vi "rsscope_FormatUSBPDPacketTypeInt32_WriteCallback.vi"(5 "Attribute":T1={"Identifier"="", "Descriptive Name"="", "Data Type"=enum."Integer 32", "Command"="", "Access"=enum."Read/Write", "Range Table"="", "Read Callback"="", "Write Callback"="", "Supported Models"="", "Instrument Options"="", "Index"=0, "OPC Wait"=FALSE, "No Status Check"=FALSE, "Cache Only"=FALSE}, 7 "Repeated Capability":string, 8 "error in (no error)":errorcluster, 10 "Attribute Value I32":i32, 11 "VISA resource name":refnum<visa-resource-name>) -> (0 "error out":errorcluster, 3 "VISA resource name out":refnum<visa-resource-name>)   [LabVIEW 2018]
doc: "This VI sets the attribute value.\n\nThis is a low-level VI that you can use to set the values of instrument-specific properties and inherent IVI properties. If the property represents an instrument state, this VI performs instrument I/O in the following cases:\n\n- State caching is disabled for the entire session or for the particular property.\n\n- State caching is enabled and the currently cached value is invalid or is different than the value you specify. \n\nThis instrument driver contains high-level VIs that set most of the instrument properties. It is best to use the high-level driver VIs as much as possible. They handle order dependencies and multithread locking for you. In addition, they perform status checking only after setting all of the properties. In contrast, when you set multiple properties using the SetAttribute VIs, the VIs check the instrument status after each call.\n\nAlso, when state caching is enabled, the high-level VIs that configure multiple properties perform instrument I/O only for the properties whose value you change. Thus, you can safely call the high-level VIs without the penalty of redundant instrument I/O."
uses:
  rsidr_core.llb/type_Attribute.ctl
  rsidr_core.llb/type_Attribute_Data_Type.ctl
  rsidr_core.llb/type_ReadWriteAccess.ctl
  rsidr_core.llb/rsscope_rsidr_core.lvlib
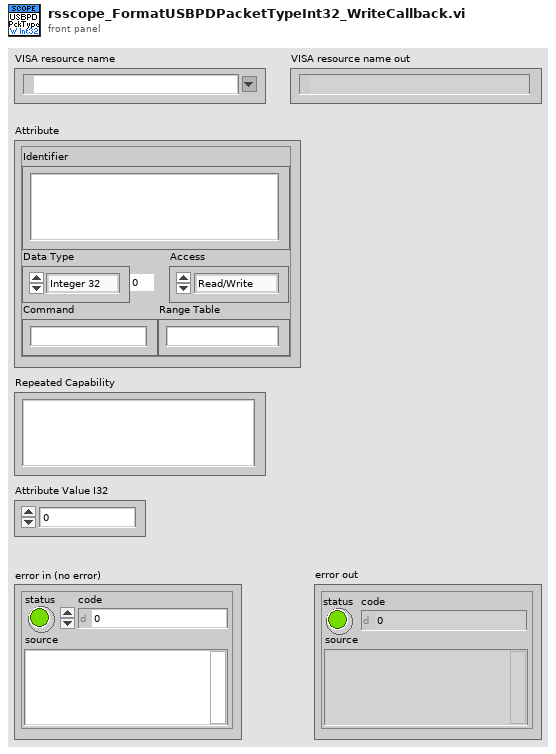
[diagram p1: front panel]
types:
  T1 = typedef "rsscope_rsidr_core.lvlib/type_Attribute.ctl" = cluster{"Identifier":string, "Descriptive Name":string, "Data Type":T2, "Command":string, "Access":T3, "Range Table":string, "Read Callback":string, "Write Callback":string, "Supported Models":string, "Instrument Options":string, "Index":i32, "OPC Wait":bool, "No Status Check":bool, "Cache Only":bool}
  T2 = typedef "rsscope_rsidr_core.lvlib/type_Attribute_Data_Type.ctl" = enum16{"Integer 32", "Double", "String", "Boolean", "None", "Integer 64", "RawString"}
  T3 = typedef "rsscope_rsidr_core.lvlib/type_ReadWriteAccess.ctl" = enum16{"Read Only", "Write Only", "Read/Write"}
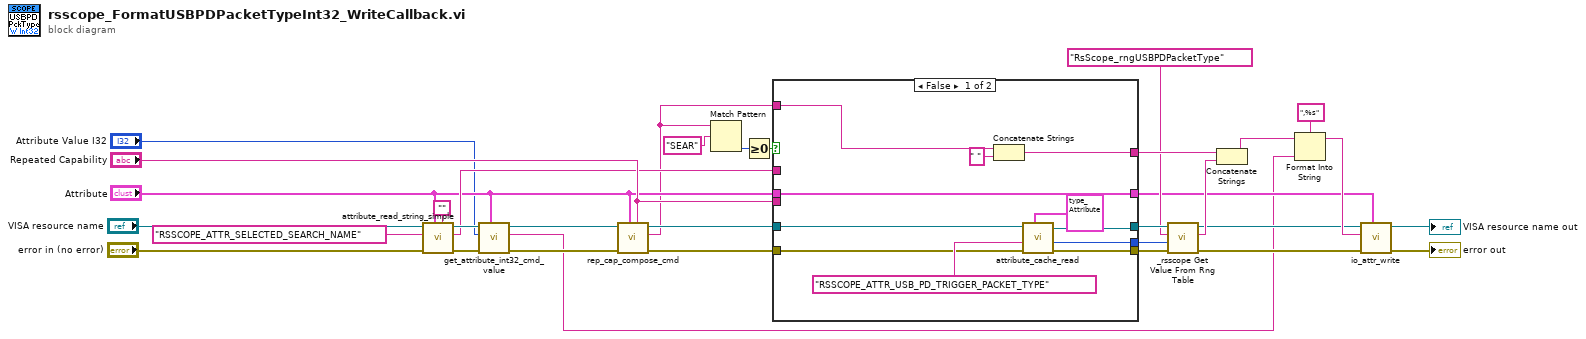
[diagram p0: block diagram]
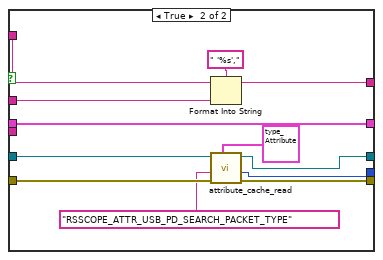
[diagram p2: hidden frame]
diagram:
  n1 = call "attribute_read_string_simple.vi"("Repeated Capability"="" ("Empty String Constant"), "Attribute"="Attribute", "error in"="error in (no error)", "Direct Attribute ID (\"\")"="RSSCOPE_ATTR_SELECTED_SEARCH_NAME" ("Direct Attribute ID (\"\")"), "VISA resource name"="VISA resource name") -> ("error out"=w27:errorcluster, "String out"=w8:string, "VISA resource name out"=w26:refnum<visa-resource-name>)  [unwired: 4 in]
  n2 = call "get_attribute_int32_cmd_value.vi"("Attribute"="Attribute", "error in"=w27, "Input Int32 value"="Attribute Value I32", "VISA resource name"=w26) -> ("error out"=w25:errorcluster, "Cmd Value out"=w1:string, "VISA resource name out"=w24:refnum<visa-resource-name>)  [unwired: 5 in]
  n3 = call "rep_cap_compose_cmd.vi"("Repeated Capability"="Repeated Capability", "Attribute"="Attribute", "error in"=w25, "VISA resource name"=w24) -> ("error out"=w13:errorcluster, "Command out"=w3:string, "VISA resource name out"=w12:refnum<visa-resource-name>)  [unwired: 5 in]
  n4 = Match Pattern(string=w3, regular expression="SEAR" ("true string")) -> (offset past match=w16:i32)  [unwired: 1 in, 3 out]
  n5 = Greater Or Equal To 0?(x=w16) -> (x >= 0?=w15:bool)
  n6 = case shown="False" w15 {
    tunnel: w8 -> [_ w55]
    tunnel: [w44 w54] -> w22
    tunnel: w3 -> [w34 w53]
    tunnel: w12 -> [w38 w49]
    tunnel: w13 -> [w39 w50]
    tunnel: [w36 w48] -> w21
    tunnel: [w37 w47] -> w20
    tunnel: [w35 w46] -> w19
    tunnel: "Repeated Capability" -> [_ _]
    tunnel: "Attribute" -> [w42 w52]
    tunnel: [w42 w52] -> w6
    frame False {
      n7 = Concatenate Strings(w34, " " ("string")) -> (w44:string)
      n8 = call "attribute_cache_read.vi"("Attribute"=T1 {"Identifier"="", "Descriptive Name"="", "Data Type"=enum."Integer 32", "Command"="", "Access"=enum."Read/Write", "Range Table"="", "Read Callback"="", "Write Callback"="", "Supported Models"="", "Instrument Options"="", "Index"=0, "OPC Wait"=FALSE, "No Status Check"=FALSE, "Cache Only"=FALSE}, "error in"=w39, "Direct Attribute ID (Attribute cluster)"="RSSCOPE_ATTR_USB_PD_TRIGGER_PACKET_TYPE" ("Direct Attribute ID (\"\")"), "VISA resource name"=w38) -> ("error out"=w37:errorcluster, "Int32 out"=w35:i32, "VISA resource name out"=w36:refnum<visa-resource-name>)  [unwired: 5 out]
    }
    frame True {
      n9 = Format Into String(format string=" '%s',", initial string=w53, w55) -> (resulting string=w54:string)  [unwired: 1 in, 1 out]
      n10 = call "attribute_cache_read.vi"("Attribute"=T1 {"Identifier"="", "Descriptive Name"="", "Data Type"=enum."Integer 32", "Command"="", "Access"=enum."Read/Write", "Range Table"="", "Read Callback"="", "Write Callback"="", "Supported Models"="", "Instrument Options"="", "Index"=0, "OPC Wait"=FALSE, "No Status Check"=FALSE, "Cache Only"=FALSE}, "error in"=w50, "Direct Attribute ID (Attribute cluster)"="RSSCOPE_ATTR_USB_PD_SEARCH_PACKET_TYPE" ("Direct Attribute ID (\"\")"), "VISA resource name"=w49) -> ("error out"=w47:errorcluster, "Int32 out"=w46:i32, "VISA resource name out"=w48:refnum<visa-resource-name>)  [unwired: 5 out]
    }
  }
  n11 = call "_rsscope Get Value From Rng Table.vi"("error in (no error)"=w20, "Value"=w19, "Range Table Name"="RsScope_rngUSBPDPacketType", "VISA resource name"=w21) -> ("error out"=w10:errorcluster, "Output Enum value"=w17:string, "VISA resource name out"=w11:refnum<visa-resource-name>)  [unwired: 5 in]
  n12 = Concatenate Strings(w22, w17) -> (w5:string)
  n13 = Format Into String(format string=",%s", initial string=w5, w1) -> (resulting string=w23:string)  [unwired: 1 in, 1 out]
  n14 = call "io_attr_write.vi"("Attribute"=w6, "error in"=w10, "write buffer"=w23, "VISA resource name"=w11) -> ("error out"=→"error out":errorcluster, "VISA resource name out"=→"VISA resource name out":refnum<visa-resource-name>)  [unwired: 6 in]
